vi "CSC_GetCableInGCS.vi"(8 "error in (no error)":errorcluster, 11 "C-Alex in":refnum<class "CableSerialChain.lvclass">) -> (0 "error out":errorcluster, 2 "Cables Points":cluster{"PointInGCS":dbl[][]}[](array[cluster]), 3 "C-Alex out":refnum<class "CableSerialChain.lvclass">)   [LabVIEW 2015, in "CableSerialChain.lvclass"]
uses:
  CableSerialChain.lvclass
  CableSerialChain.lvclass/CableSerialChain.ctl
  <vilib>/Analysis/BLAS.llb/gemv - General Matrix-Vector Product.vi
  <vilib>/Analysis/BLAS.llb/dgemv - General Matrix-Vector Product (DBL).vi
  <vilib>/Utility/error.llb/Error Cluster From Error Code.vi
  Body/Bodies.lvclass
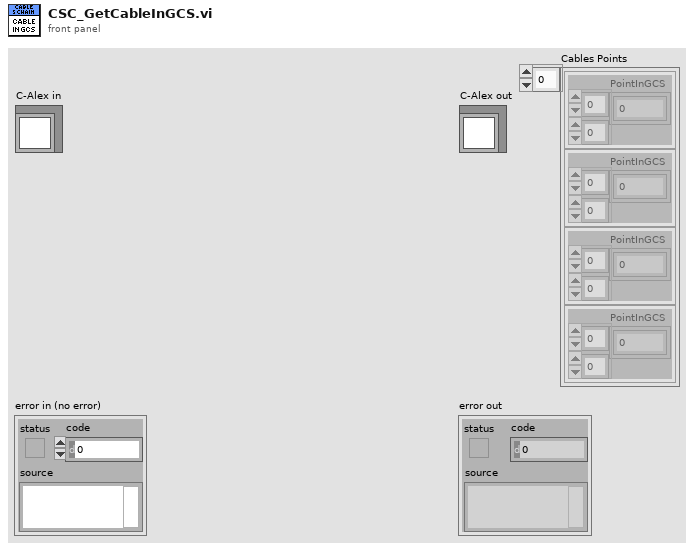
[diagram p1: front panel]
types:
  T1 = typedef "CableSerialChain.lvclass/Cable.ctl" = cluster{"RoutingPtsInLCS":T2[], "Cable ID":i32, "ActiveSegments":i32[][]}
  T2 = typedef "Bodies.lvclass/PointOnBody.ctl" = cluster{"Coord4":dbl[], "ID":i32}
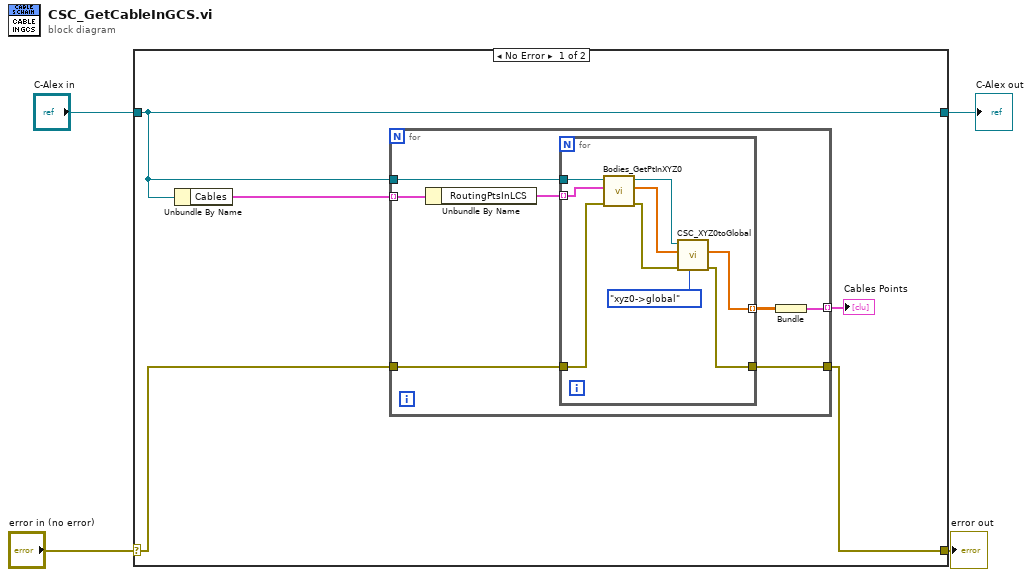
[diagram p0: block diagram]
diagram:
  n1 = case shown="No Error" "error in (no error)" {
    selector: "error in (no error)" -> [w7 w26]
    tunnel: [w5 w27] -> w2
    tunnel: "C-Alex in" -> [w5 w27]
    tunnel: [w6 w26] -> w1
    frame No Error {
      n2 = Unbundle By Name(w5) -> ("Cables"=w8:T1[])
      n3 = for {
        tunnel: w8 -> [w16] mode=indexing
        tunnel: [w12] -> w9 mode=indexing
        tunnel: w5 -> [w15]
        tunnel: w7 -> [w11]
        tunnel: [w10] -> w6
        n4 = Unbundle By Name(w16) -> ("RoutingPtsInLCS"=w14:T2[])
        n5 = for {
          tunnel: w14 -> [w24] mode=indexing
          tunnel: [w22] -> w13 mode=indexing
          tunnel: w15 -> [w25]
          tunnel: w11 -> [w20]
          tunnel: [w21] -> w10
          n6 = call "Bodies_GetPtInXYZ0.vi"("error in (no error)"=w20, "Point"=w24, "Bodies.lvclass"=w25) -> ("error out"=w19:errorcluster, "PointInGCS"=w23:dbl[], "Bodies.lvclass 2"=w17:refnum<class "CableSerialChain.lvclass">)  [unwired: 5 in, 1 out]
          n7 = call "CSC_XYZ0toGlobal.vi"("Dir(xyz0->global)"=enum16{"global->xyz0", "xyz0->global"}."xyz0->global", "error in (no error)"=w19, "Pin"=w23, "CSC In"=w17) -> ("error out"=w21:errorcluster, "Pout"=w22:dbl[])  [unwired: 4 in, 2 out]
        }
        n8 = Bundle("Pout"=w13) -> (w12:cluster{"Pout":dbl[][]})  [unwired: 1 in]
      }
      "Cables Points" <- w9
    }
    frame Error {
    }
  }
  "error out" <- w1
  "C-Alex out" <- w2
